vi "ShiftRegisterForLoop.vi"() -> ()   [LabVIEW 2020]
panel:
  out "Numeric":dbl
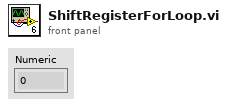
[diagram p1: front panel]
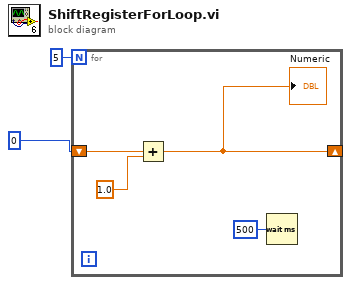
[diagram p0: block diagram]
diagram:
  n1 = for {
    N: 5 -> [_]
    shift-right: [w4] -> _
    shift-left: 0 -> [w5]
    n2 = Add(x=w5, y=1.0) -> (x+y=w4:dbl)
    "Numeric" <- w4
    n3 = Wait (ms)(milliseconds to wait=u32 500) -> ()  [unwired: 1 out]
  }
